vi "Math-Uniform Random Number (I32, scalar).vi"(4 "Ymax":i32, 5 "Ymin":i32) -> (1 "Random Int":i32)   [LabVIEW 2020]
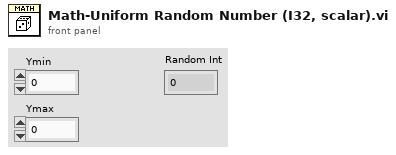
[diagram p1: front panel]
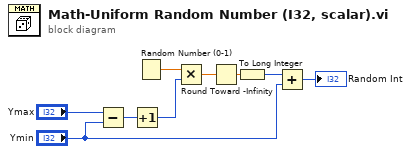
[diagram p0: block diagram]
diagram:
  n1 = Subtract(x="Ymax", y="Ymin") -> (x-y=w6:i32)
  n2 = Increment(x=w6) -> (x+1=w5:i32)
  n3 = Random Number (0-1)() -> (number: 0 to 1=w9:dbl)
  n4 = Multiply(x=w9, y=w5) -> (x*y=w8:dbl)
  n5 = Round Toward -Infinity(1:w8) -> (0:w7:dbl)
  n6 = To Long Integer(number=w7) -> (32bit integer=w4:i32)
  n7 = Add(x=w4, y="Ymin") -> (x+y=→"Random Int":i32)
